vi "AgPSA _Set Freq and Acquire Peak.vi"(6 "Route Names":string[](array[string]), 8 "error in (no error)":errorcluster, 9 "Span(Hz)":dbl=26500000000.0, 10 "Center Frequency(Hz)":u64=13250000000, 11 "VISA resource name":refnum<visa-resource-name>) -> (0 "error out":errorcluster, 1 "Amplitude (Cal)":dbl, 2 "Frequency":dbl format="%#_6f", 3 "VISA out":refnum<visa-resource-name>, 4 "FDelta":dbl)   [LabVIEW 2015]
uses:
  <instrlib>/Agilent MXA Series/Public/Configure/Configure Frequency (Center Span).vi
  <instrlib>/Agilent MXA Series/Agilent MXA Series.lvlib
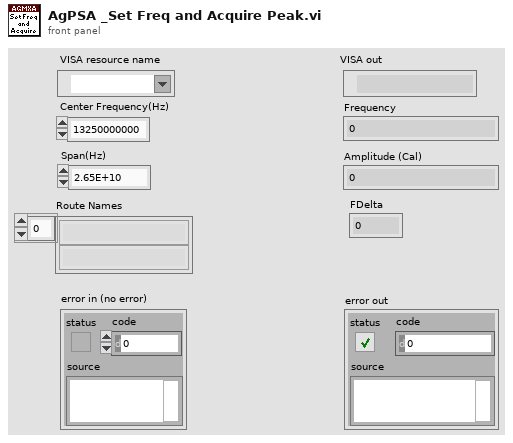
[diagram p1: front panel]
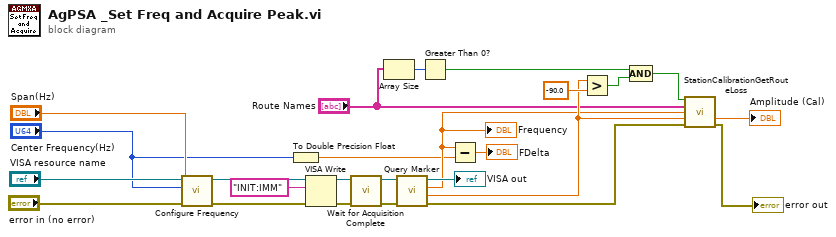
[diagram p0: block diagram]
diagram:
  n1 = call-poly <instrlib>:"Configure Frequency.vi"("error in (no error)"="error in (no error)", "Span (2.65E+10 Hz)"="Span(Hz)", "Center Frequency (1.325E+10 Hz)"="Center Frequency(Hz)", "VISA resource name"="VISA resource name") -> ("error out"=w19:errorcluster, "VISA resource name out"=w21:refnum<visa-resource-name>)  [unwired: 6 in]
  n2 = To Double Precision Float(number="Center Frequency(Hz)") -> (double precision float=w1:dbl)
  n3 = VISA Write(VISA resource name=w21, write buffer="INIT:IMM" ("format string"), error in (no error)=w19) -> (VISA resource name out=w18:refnum<visa-resource-name>, error out=w16:errorcluster)  [unwired: 1 out]
  n4 = call <instrlib>:"Wait for Acquisition Complete.vi"("error in (no error)"=w16, "VISA resource name"=w18) -> ("error out"=w15:errorcluster, "VISA resource name out"=w17:refnum<visa-resource-name>)  [unwired: 8 in]
  n5 = Array Size(array="Route Names") -> (size(s)=w8:i32)
  n6 = call <instrlib>:"Query Marker.vi"("error in (no error)"=w15, "VISA resource name"=w17) -> ("error out"=w11:errorcluster, "Marker Amplitude"=w12:dbl, "Marker Position"=w4:dbl, "VISA resource name out"=→"VISA out":refnum<visa-resource-name>)  [unwired: 6 in]
  "Frequency" <- w4
  n7 = Greater Than 0?(x=w8) -> (x > 0?=w5:bool)
  n8 = Subtract(x=w4, y=w1) -> (x-y=→"FDelta":dbl)
  n9 = Greater?(x=w12, y=-90.0) -> (0:w7:bool)
  n10 = Compound Arithmetic op=AND(w5, w7) -> (w6:bool)
  n11 = call "StationCalibrationGetRouteLoss.vi"("Calibration Enabled"=w6, "Route Names"="Route Names", "Frequency"=w4, "Power Level"=w12, "error in (no error)"=w11) -> ("Adjusted Power Level"=→"Amplitude (Cal)":dbl, "error out"=→"error out":errorcluster)  [unwired: 7 in, 2 out]
